vi "Close.vi"(8 "error in (no error)":errorcluster, 11 "navX - Base in":refnum<class "navX - Base.lvclass">) -> (0 "error out":errorcluster, 3 "navX - Base out":refnum<class "navX - Base.lvclass">)   [LabVIEW 2015, in "navX Library v3.lvlib" / "navX - Base.lvclass"]
uses:
  navX - Base.lvclass
  navX - Base.lvclass/navX - Base.ctl
  navX Registry Cache/navX Registry Cache.lvclass
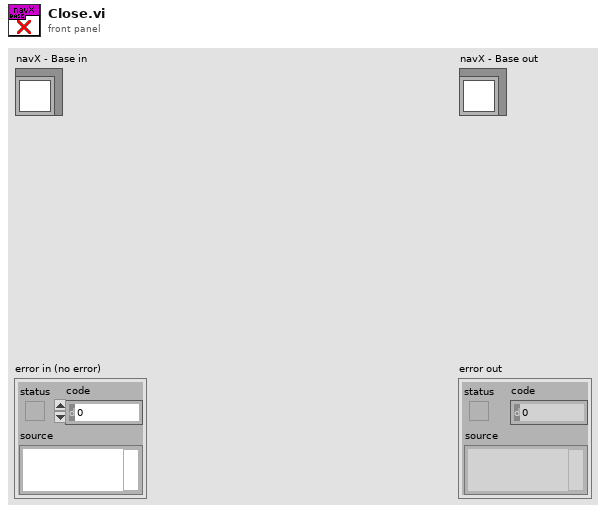
[diagram p1: front panel]
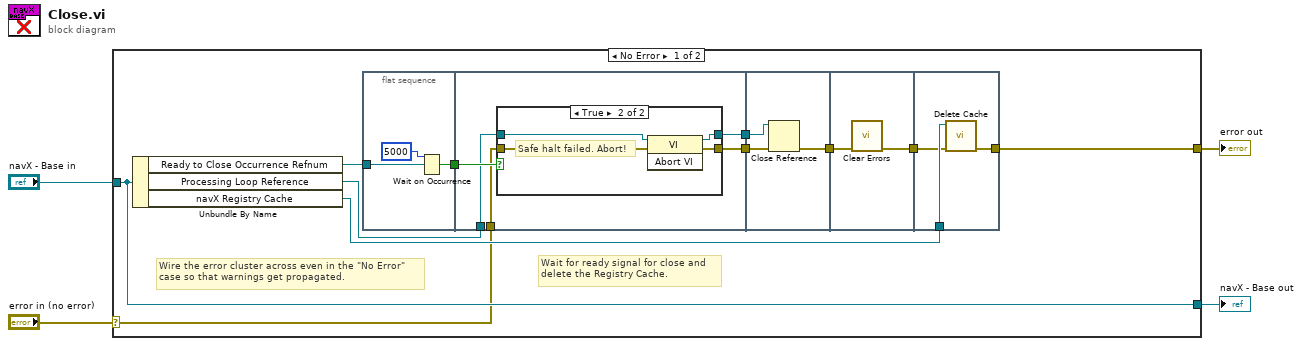
[diagram p0: block diagram]
diagram:
  n1 = case shown="No Error" "error in (no error)" {
    selector: "error in (no error)" -> [w7 w39]
    tunnel: [w14 w39] -> w3
    tunnel: [w15 w38] -> w1
    tunnel: "navX - Base in" -> [w15 w38]
    frame No Error {
      # "Wait for ready signal for close and\ndelete the Registry Cache."
      # "Wire the error cluster across even in the \"No Error\"\ncase so that warnings get propagated."
      n2 = Unbundle By Name(w15) -> ("Ready to Close Occurrence Refnum"=w9:refnum<k4>, "Processing Loop Reference"=w8:refnum<vi>, "navX Registry Cache"=w13:refnum<class "navX Registry Cache.lvclass">)
      n3 = flat-sequence {
        tunnel: w9 -> [w18]
        tunnel: [w16] -> w12
        tunnel: w12 -> [w23]
        tunnel: w8 -> [w22]
        tunnel: w7 -> [w21]
        tunnel: [w20] -> w6
        tunnel: [w19] -> w5
        tunnel: [w32] -> w11
        tunnel: w6 -> [w31]
        tunnel: w5 -> [w30]
        tunnel: w11 -> [w34]
        tunnel: [w33] -> w10
        tunnel: [w37] -> w14
        tunnel: w13 -> [w36]
        tunnel: w10 -> [w35]
        frame #0 {
          n4 = Wait on Occurrence(2:w18, 3:5000 ("ms timeout (-1)")) -> (0:w16:bool)  [unwired: 1 in]
        }
        frame #1 {
          n5 = case shown="True" w23 {
            tunnel: w22 -> [w25 w29]
            tunnel: w21 -> [w24 w28]
            tunnel: [w24 w26] -> w20
            tunnel: [w25 w27] -> w19
            frame False {
              # "Safe abort success"
            }
            frame True {
              # "Safe halt failed. Abort!"
              n6 = invoke class="VI" method="Abort VI"(reference=w29, error in=w28) -> (reference out=w27:refnum<vi>, error out=w26:errorcluster)  [unwired: 1 in, 1 out]
            }
          }
        }
        frame #2 {
          n7 = Close Reference(reference=w30, error in (no error)=w31) -> (error out=w32:errorcluster)
        }
        frame #3 {
          n8 = call <vilib>:"Clear Errors.vi"("error in (no error)"=w34) -> ("error out"=w33:errorcluster)  [unwired: 5 in, 1 out]
        }
        frame #4 {
          n9 = call "Delete Cache.vi"("error in (no error)"=w35, "navX Registry Cache in"=w36) -> ("error out"=w37:errorcluster)  [unwired: 7 in, 2 out]
        }
      }
    }
    frame Error {
    }
  }
  "error out" <- w3
  "navX - Base out" <- w1
